vi "Multiplot Graph.vi"() -> ()   [LabVIEW 2018]
panel:
  in  "Square Frequency":dbl(slide) scale=0.0..50.0
  in  "Sine Frequency":dbl(slide) scale=0.0..50.0
  in  "stop":bool
  out "Waveform Graph":dynamicdata(graph)
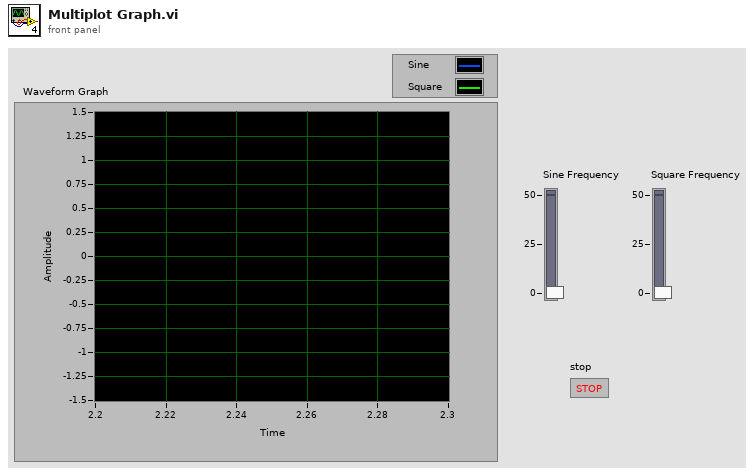
[diagram p1: front panel]
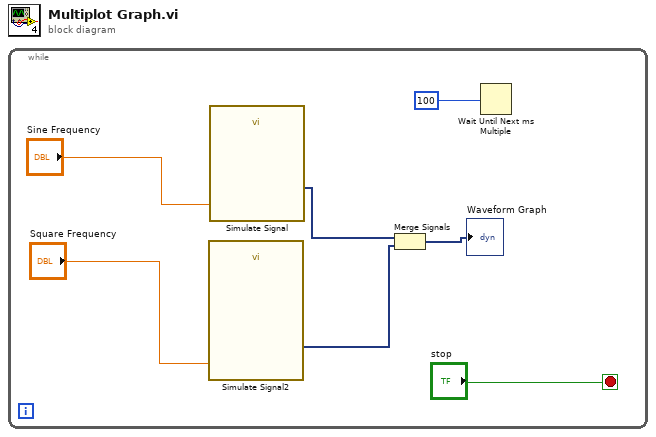
[diagram p0: block diagram]
diagram:
  n1 = while {
    stop <- "stop" stop-if-true
    n2 = call "Simulate Signal2"("Frequency"="Square Frequency") -> ("Square"=w1:dynamicdata)  [unwired: 13 in, 1 out]
    n3 = call "Simulate Signal"("Frequency"="Sine Frequency") -> ("Sine"=w3:dynamicdata)  [unwired: 13 in, 1 out]
    n4 = Merge Signals(w3, w1) -> (→"Waveform Graph":dynamicdata)
    n5 = Wait Until Next ms Multiple(millisecond multiple=u32 100 ("millisecond timer value")) -> ()  [unwired: 1 out]
  }
